vi "SandboxRunner.vi"() -> ()   [LabVIEW 2025]
uses:
  FpgaRunner/FpgaRunner.lvclass
panel:
  in  "Data":u64[](array[numeric])=[1, 2864434397, 0, 4009693474, 0, 3735928559, 2, 73588229205] format="%.0x"
  out "Array":u64[](array[numeric]) format="%.0x"
  out "error out":errorcluster
  in  "error in (no error)":errorcluster
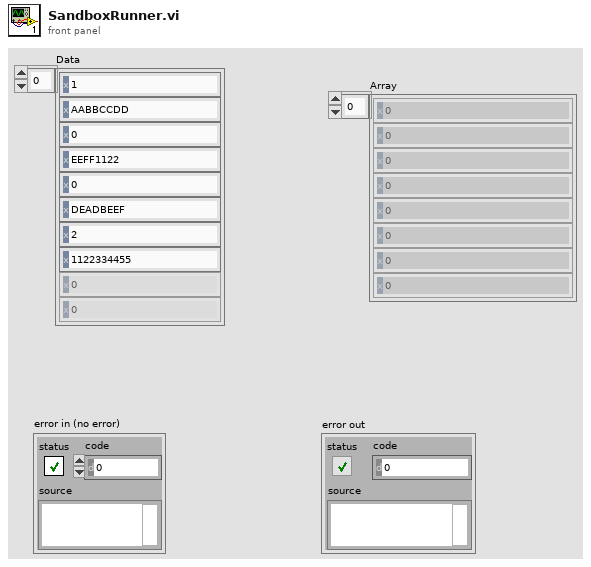
[diagram p1: front panel]
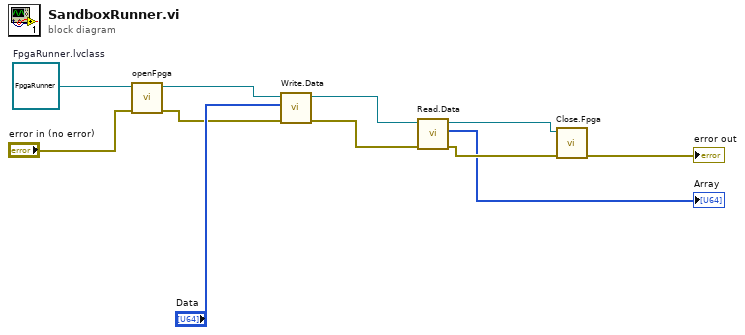
[diagram p0: block diagram]
diagram:
  w11 = refnum<class "FpgaRunner.lvclass"> refnum  # FpgaRunner.lvclass
  n1 = call-dynamic "openFpga.vi"("error in (no error)"="error in (no error)", "FpgaRunner in"=w11) -> ("error out"=w7:errorcluster, "FpgaRunner out"=w9:refnum<class "FpgaRunner.lvclass">)  [unwired: 8 in]
  n2 = call-dynamic "Write.Data.vi"("error in (no error)"=w7, "Data"="Data", "FpgaRunner in"=w9) -> ("error out"=w6:errorcluster, "FpgaRunner out"=w5:refnum<class "FpgaRunner.lvclass">)  [unwired: 7 in]
  n3 = call-dynamic "Read.Data.vi"("error in (no error)"=w6, "FpgaRunner in"=w5) -> ("error out"=w3:errorcluster, "Array"=→"Array":u64[], "FpgaRunner out"=w1:refnum<class "FpgaRunner.lvclass">)  [unwired: 7 in]
  n4 = call-dynamic "Close.Fpga.vi"("error in (no error)"=w3, "FpgaRunner in"=w1) -> ("error out"=→"error out":errorcluster)  [unwired: 8 in, 1 out]
